vi "DP-Init DataAcq.vi"(0 "StimGen":T2, 1 "Expt State":T4, 5 "DP stimulus params":T1={"Ear"=enum."Left", "f2 freqs (kHz)"="", "Start (dB)"=20.0, "Stop (dB)"=80.0, "Step (dB)"=10.0, "Mode"=enum."L1 = L2", "override recal"=FALSE, "Sampling Rate (Hz)"=0.0, "Frame (ms)"=0}, 7 "Init data file (T)":bool=TRUE, 9 "Avg specs":T5={"# time avgs "=8, "# spectra avgs"=4}, 11 "error in (no error)":errorcluster, 12 "Mic gain (dB)":dbl, 13 "Save waves?":bool) -> (3 "Expt State out":T4, 4 "DataAcq":T3, 6 "DP thru":T1={"Ear"=enum."Left", "f2 freqs (kHz)"="", "Start (dB)"=20.0, "Stop (dB)"=80.0, "Step (dB)"=10.0, "Mode"=enum."L1 = L2", "override recal"=FALSE, "Sampling Rate (Hz)"=0.0, "Frame (ms)"=0}, 15 "error out":errorcluster)   [LabVIEW 2020]
uses:
  Misc VIs/Connection Manager/Type Defs/Input sources.ctl
  Typedefs/DP Stimulus Params.ctl
  CFTS SubVIs/CFTS-Experiment State.ctl
  Typedefs/DP-DataAcq.ctl
  Typedefs/DP-StimGen.ctl
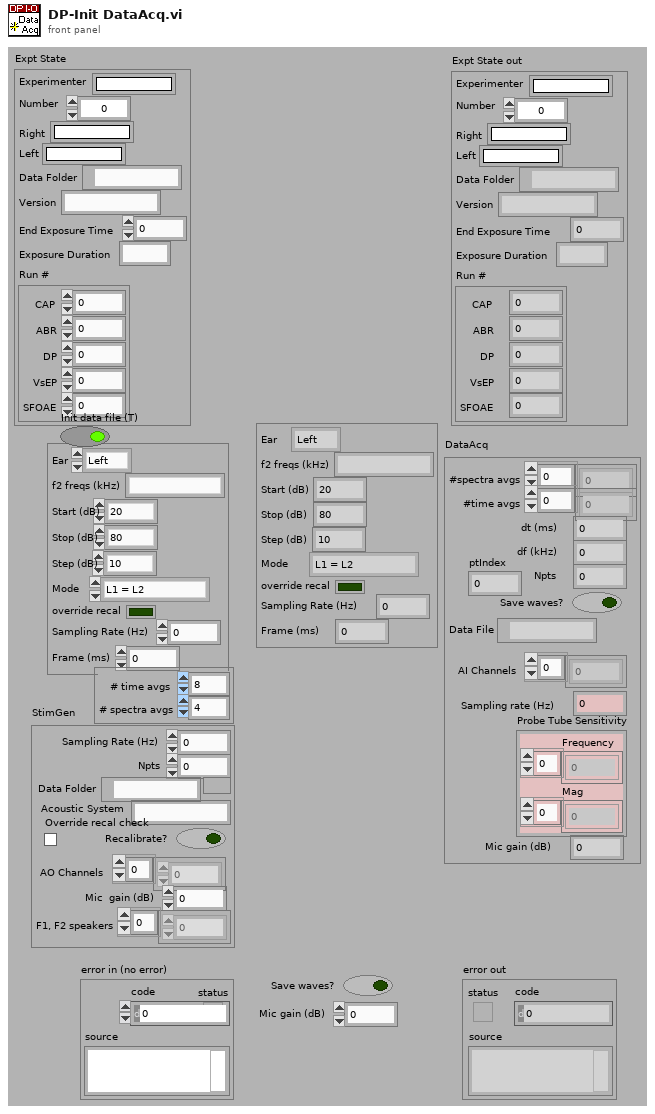
[diagram p1: front panel]
types:
  T1 = typedef "DP Stimulus Params.ctl" = cluster{"Ear":enum16{"Right", "Left"}, "f2 freqs (kHz)":string, "Start (dB)":dbl, "Stop (dB)":dbl, "Step (dB)":dbl, "Mode":enum16{"L1 = L2", "L1 = L2 + 10 dB"}, "override recal":bool, "Sampling Rate (Hz)":dbl, "Frame (ms)":i32}
  T2 = typedef "DP-StimGen.ctl" = cluster{"Sampling Rate (Hz)":dbl, "Npts":i32, "Data Folder":path, "Acoustic System":string, "Recalibrate?":bool, "AO Channels":i32[], "Mic  gain (dB)":dbl, "F1, F2 speakers":i32[], "Override recal check":bool}
  T3 = typedef "DP-DataAcq.ctl" = cluster{"#spectra avgs":i32[], "#time avgs":i32[], "dt (ms)":dbl, "df (kHz)":dbl, "Npts":i32, "Save waves?":bool, "Data File":path, "AI Channels":u16[], "Sampling rate (Hz)":dbl, "Probe Tube Sensitivity":cluster{"Frequency":dbl[], "Mag":dbl[]}, "Mic gain (dB)":dbl, "ptIndex":i32}
  T4 = typedef "CFTS-Experiment State.ctl" = cluster{"Experimenter":string, "Number":u32, "Right":string, "Left":string, "Data Folder":path, "Version":string, "End Exposure Time":dbl, "Exposure Duration":string, "Run #":cluster{"CAP":i32, "ABR":i32, "DP":i32, "VsEP":i32, "SFOAE":i32}}
  T5 = cluster{"# time avgs ":i32, "# spectra avgs":i32}
  T6 = typedef "Input sources.ctl" = u16
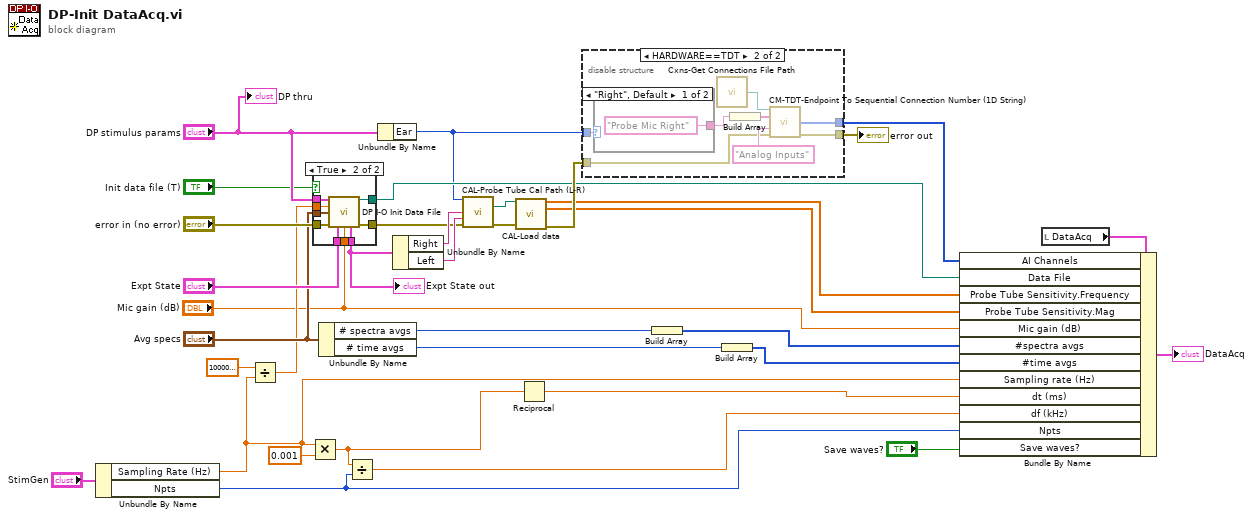
[diagram p0: block diagram]
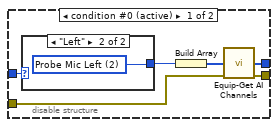
[diagram p2: hidden frame]
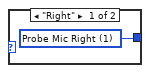
[diagram p3: hidden frame]
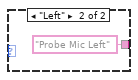
[diagram p4: hidden frame]
diagram:
  n1 = Unbundle By Name("StimGen") -> ("Sampling Rate (Hz)"=w7:dbl, "Npts"=w6:i32)
  n2 = Divide(x=1000000.0, y=w7) -> (x/y=w11:dbl)
  n3 = Multiply(x=w7, y=0.001 ("x")) -> (x*y=w10:dbl)
  n4 = case shown="True" "Init data file (T)" {
    tunnel: "error in (no error)" -> [w37 w46]
    tunnel: "DP stimulus params" -> [_ w45]
    tunnel: "Expt State" -> [w36 w44]
    tunnel: [w37 w43] -> w30
    tunnel: [w36 w42] -> w25
    tunnel: [_ w41] -> w19
    tunnel: "Avg specs" -> [_ w40]
    tunnel: w11 -> [_ w39]
    tunnel: "Mic gain (dB)" -> [_ w38]
    frame False {
    }
    frame True {
      n5 = call "DP I-O Init Data File.vi"("DP stimulus params"=w45, "Sampling interval (us)"=w39, "Averaging Specs"=w40, "error in (no error)"=w46, "Expt State"=w44, "Probe Mic Gain (dB)"=w38) -> ("Path"=w41:path, "Expt State out"=w42:T4, "error out"=w43:errorcluster)  [unwired: 7 in]
    }
  }
  "Expt State out" <- w25
  n6 = Unbundle By Name("Avg specs") -> ("# spectra avgs"=w16:i32, "# time avgs"=w15:i32)
  n7 = Divide(x=w10, y=w6) -> (x/y=w13:dbl)
  n8 = Unbundle By Name("DP stimulus params") -> ("Ear"=w1:enum16{"Right", "Left"})
  n9 = Unbundle By Name(w25) -> ("Right"=w32:string, "Left"=w31:string)
  n10 = call "CAL-Probe Tube Cal Path (L-R).vi"("Ear"=w1, "Right"=w32, "Left"=w31, "error in (no error)"=w30) -> ("Probe Tube Cal Path"=w28:path, "error out"=w29:errorcluster)  [unwired: 10 in]
  n11 = call "CAL-Load data.vi"("user path"=w28, "error in (no error)"=w29) -> ("Frequency (Hz)"=w22:dbl[], "Mag"=w21:dbl[], "error out"=w24:errorcluster)  [unwired: 6 in, 5 out]
  n12 = Reciprocal(x=w10) -> (1/x=w9:dbl)
  n13 = disable-structure shown="HARDWARE==TDT" {
    disable-tunnel: w1 -> [w50 w56]
    disable-tunnel: w24 -> [w49 w58]
    disable-tunnel: [w48 w59] -> w23
    disable-tunnel: [w47 w61] -> w20
    frame condition #0 (active) {
      n14 = case shown="\"Left\"" w50 {
        tunnel: [w53 w54] -> w52
        frame "Right" {
          w53 = T6 1 items=["--unused--", "Probe Mic Right", "Probe Mic Left", "Cal Mic", "ABR", "CAP Right", "CAP Left", "Startle piezo", "Temperature", "Heart rate"] ("Ring")
        }
        frame "Left" {
          w54 = T6 2 items=["--unused--", "Probe Mic Right", "Probe Mic Left", "Cal Mic", "ABR", "CAP Right", "CAP Left", "Startle piezo", "Temperature", "Heart rate"] ("Ring")
        }
      }
      n15 = Build Array(w52) -> (w51:T6[])
      n16 = call "Equip-Get AI Channels.vi"("Inputs"=w51, "error in (no error)"=w49) -> ("AI Channels"=w47:i32[], "error out"=w48:errorcluster)  [unwired: 12 in]
    }
    frame condition #1 {
      n17 = case shown="\"Right\", Default" w56 {
        tunnel: ["Probe Mic Right" "Probe Mic Left"] -> w55
        frame "Right", Default {
        }
        frame "Left" {
        }
      }
      n18 = call "Cxns-Get Connections File Path.vi"() -> ("Path Out"=w60:path)  [unwired: 1 in]
      n19 = Build Array(w55) -> (w57:string[])
      n20 = call "CM-TDT-Endpoint To Sequential Connection Number (1D String).vi"("Path In"=w60, "Endpoints"=w57, "Section"="Analog Inputs", "error in (no error)"=w58) -> ("SeqCxnNum"=w61:i32[], "error out"=w59:errorcluster)  [unwired: 9 in, 1 out]
    }
  }
  "error out" <- w23
  n21 = Build Array(w16) -> (w3:i32[])
  n22 = Build Array(w15) -> (w2:i32[])
  n23 = local read "DataAcq"() -> (w27:T3)
  n24 = Bundle By Name(cluster=w27, "AI Channels"=w20, "Data File"=w19, "Probe Tube Sensitivity.Frequency"=w22, "Probe Tube Sensitivity.Mag"=w21, "Mic gain (dB)"="Mic gain (dB)", "#spectra avgs"=w3, "#time avgs"=w2, "Sampling rate (Hz)"=w7, "dt (ms)"=w9, "df (kHz)"=w13, "Npts"=w6, "Save waves?"="Save waves?") -> (→"DataAcq":T3)
  "DP thru" <- "DP stimulus params"
